vi "Sgl_SetProperty.vi"(1 "Property":dbl, 5 "error in (no error)":errorcluster) -> (19 "error out":errorcluster)   [LabVIEW 2012, in "SingletonTemplate.lvclass"]
uses:
  <resource>/Framework/Providers/Open_GDS/ClassProviders/Provider_EndevoGOOP300/Templates/SingletonTemplate/SingletonTemplate.lvclass
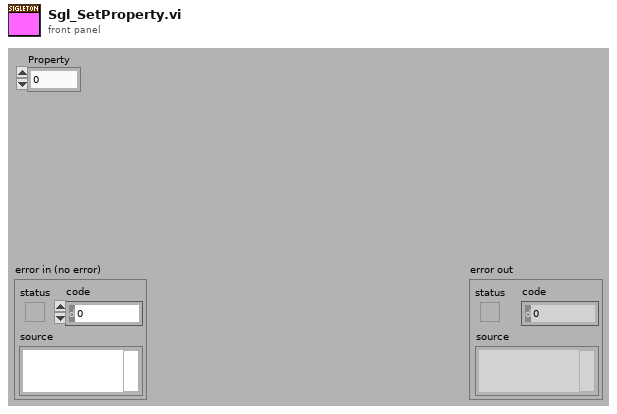
[diagram p1: front panel]
types:
  T1 = typedef "SingletonTemplate.lvclass/ObjectAttributes.ctl" = cluster{"Attribute1":dbl}
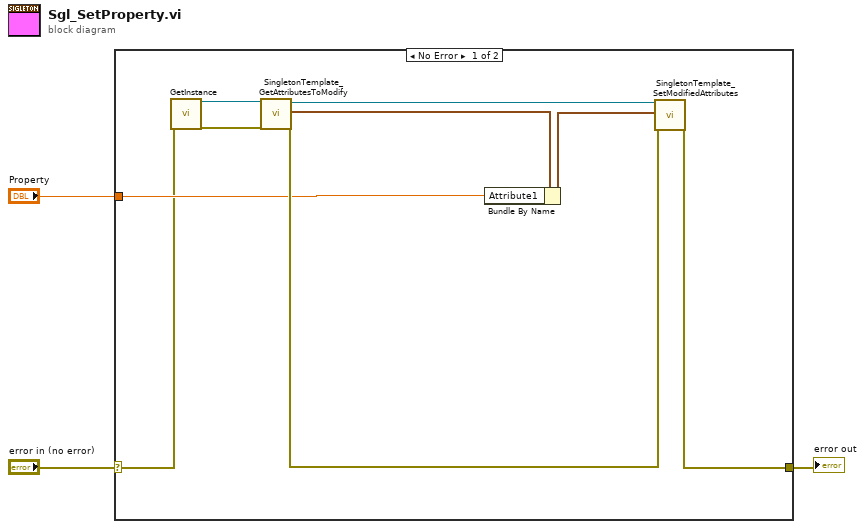
[diagram p0: block diagram]
diagram:
  n1 = case shown="No Error" "error in (no error)" {
    selector: "error in (no error)" -> [w4 w13]
    tunnel: [w9 w13] -> w2
    tunnel: "Property" -> [w7 _]
    frame No Error {
      n2 = call <resource>:"GetInstance.vi"("error in (no error)"=w4) -> ("reference out"=w5:refnum<class "SingletonTemplate.lvclass">, "error out"=w6:errorcluster)  [unwired: 17 in]
      n3 = call <resource>:"SingletonTemplate_GetAttributesToModify.vi"("reference in"=w5, "error in (no error)"=w6) -> ("reference out"=w10:refnum<class "SingletonTemplate.lvclass">, "Attributes"=w12:T1, "error out"=w8:errorcluster)  [unwired: 14 in, 1 out]
      n4 = Bundle By Name(cluster=w12, "Attribute1"=w7) -> (w11:T1)
      n5 = call <resource>:"SingletonTemplate_SetModifiedAttributes.vi"("reference in"=w10, "Attributes"=w11, "error in (no error)"=w8) -> ("error out"=w9:errorcluster)  [unwired: 15 in, 1 out]
    }
    frame Error {
    }
  }
  "error out" <- w2
